vi "AMC Multiple Targets Example 1.vi"() -> ()   [LabVIEW 2013]
uses:
  <vilib>/NI/Tools/Keyed Array/KeyedArray.ctl
  <vilib>/NI/Tools/Keyed Array/Map String.vi
  <vilib>/NI/Tools/String/Get Case Matching.vi
  vi.lib/NI/AMC/AMC.lvlib
  <vilib>/NI/Tools/Keyed Array/Tools_KeyedArray.lvlib
panel:
  out "App Response":string
  in  "request":bool
  in  "App Request":string
  in  "Local UDP Port":u16=8000
  in  "Target UDP Port":u16=9000
  in  "Servers":i32(listbox)
  in  "Get All Queues":bool
  in  "Target IP Address":string="localhost"
  in  "Queue":string
  in  "Verify Queue":bool
  in  "PingAll":bool
  out "Response":string
  in  "Ping":bool
  in  "Remote Exit":bool
  out "Process":bool
  in  "Remote Process":bool
  out "Status":string
  in  "Local Process":bool
  in  "Local Exit":bool
  in  "State Variables":T1
  # "Target 1"
  # "Local Messages >>"
  # "Remote Messages >>"
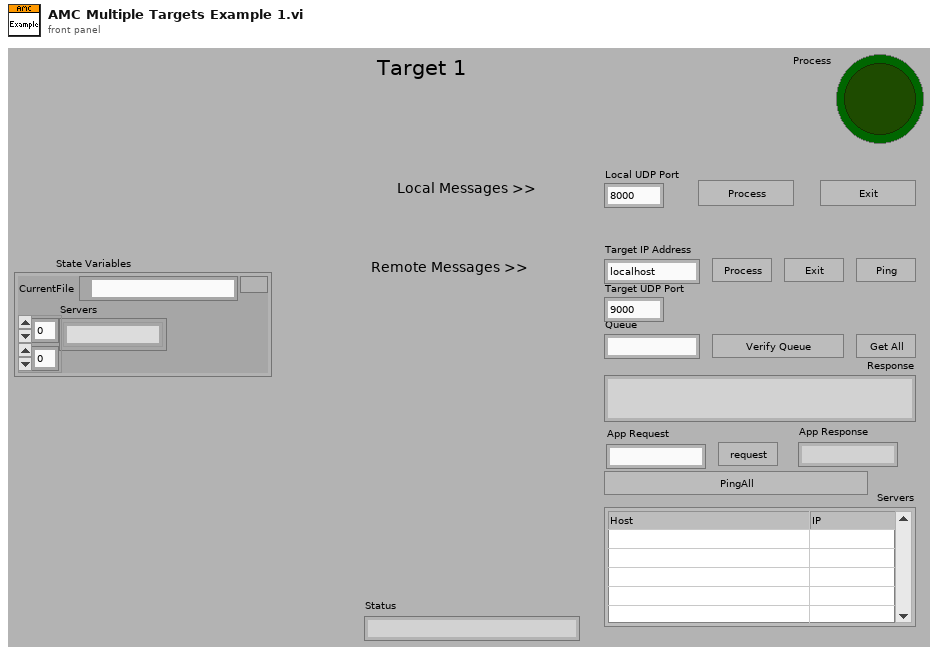
[diagram p1: front panel]
types:
  T1 = cluster{"CurrentFile":path, "Servers":string[][]}
  T2 = typedef "AMC.lvlib/Message Queue.ctl" = refnum<queue>
  T3 = typedef "AMC.lvlib/Message.ctl" = cluster{"name":string, "value":string, "attributes":T4, "receiver host":string, "receiver process":string, "source host":string, "source process":string, "priority message":bool, "acknowledge message":bool}
  T4 = typedef "Tools_KeyedArray.lvlib/KeyedArray.ctl" = cluster{"keys":string[], "values":string[]}
  T5 = typedef "LVPoint32TypeDef.ctl" = cluster{"Horizontal":i32, "Vertical":i32}
  T6 = typedef "LVRowAndColumnTypeDef.ctl" = cluster{"Row":i32, "Column":i32}
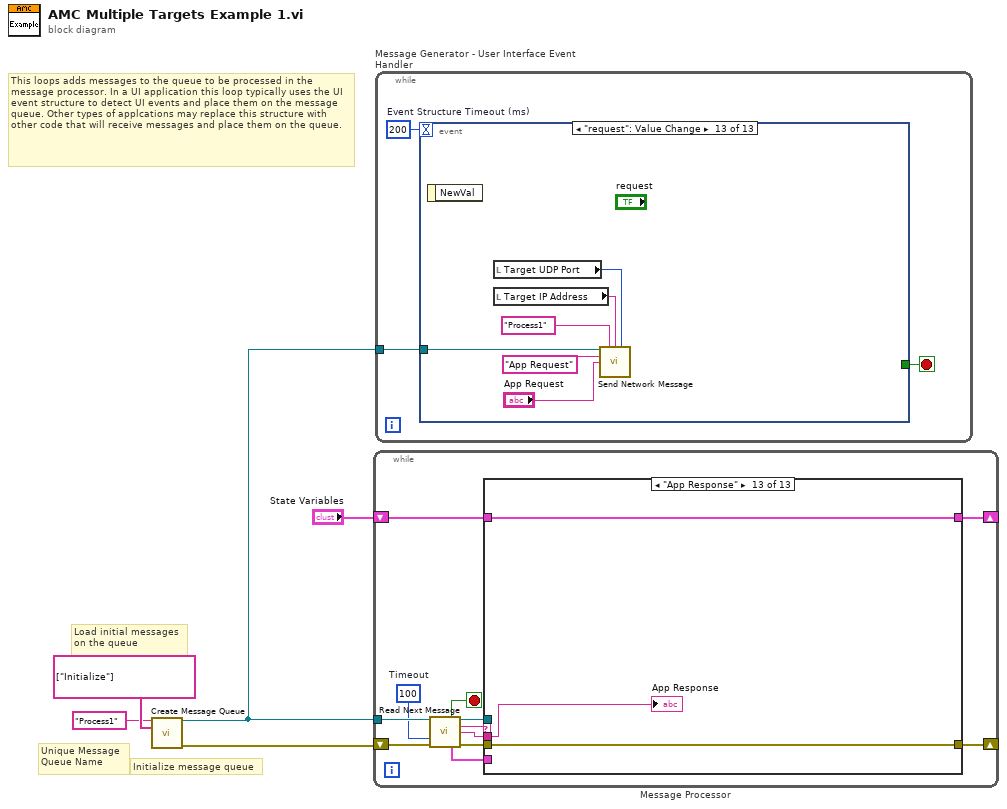
[diagram p0: block diagram]
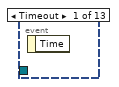
[diagram p2: hidden frame]
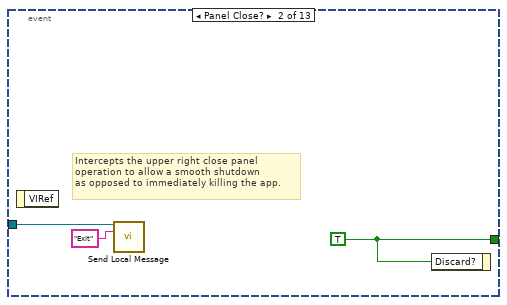
[diagram p3: hidden frame]
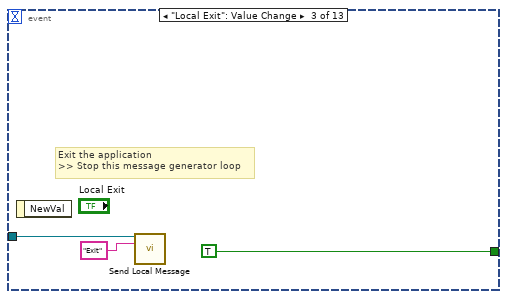
[diagram p4: hidden frame]
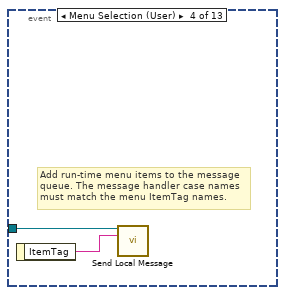
[diagram p5: hidden frame]
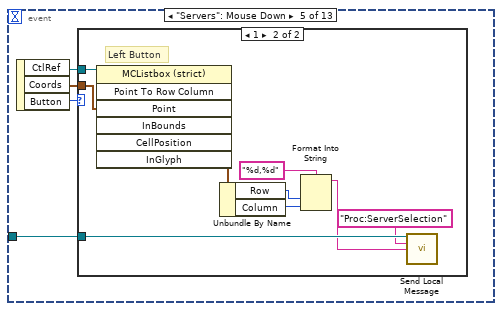
[diagram p6: hidden frame]
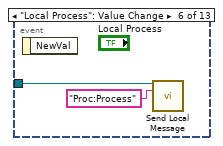
[diagram p8: hidden frame]
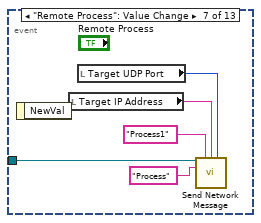
[diagram p9: hidden frame]
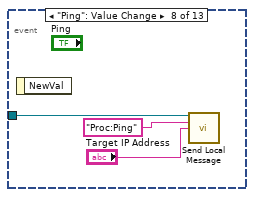
[diagram p10: hidden frame]
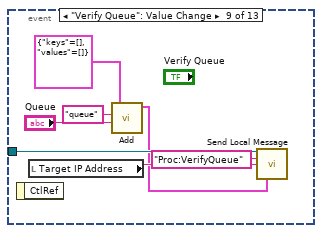
[diagram p11: hidden frame]
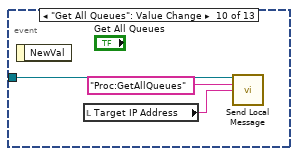
[diagram p12: hidden frame]
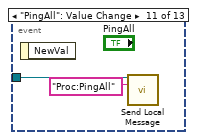
[diagram p13: hidden frame]
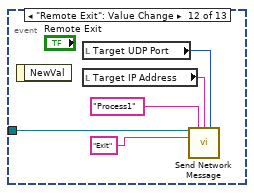
[diagram p14: hidden frame]
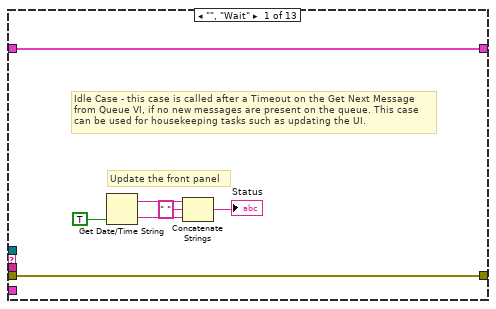
[diagram p15: hidden frame]
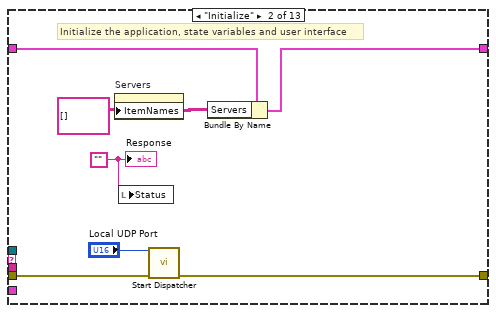
[diagram p16: hidden frame]
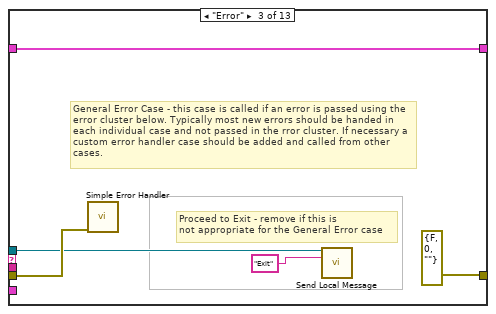
[diagram p17: hidden frame]
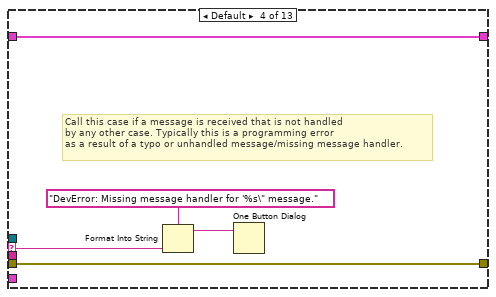
[diagram p18: hidden frame]
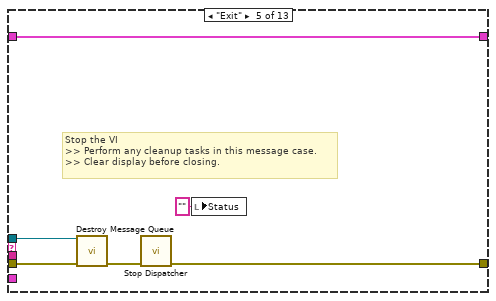
[diagram p19: hidden frame]
diagram:
  # "This loops adds messages to the queue to be processed in the message processor. In a UI application this loop typically uses the UI event structure to detect UI events and place them on the message queue. Other types of applcations may replace this structure with other code that will receive messages and place them on the queue."
  # "Initialize message queue"
  # "Unique Message\nQueue Name"
  # "Load initial messages\non the queue"
  n1 = call "Create Message Queue.vi"("message queue name"="Process1" ("Message queue name (unnamed)"), "initial message names"=string[] ["Initialize"]) -> ("message queue out"=w5:T2, "error out"=w3:errorcluster)  [unwired: 12 in]
  n2 = while "Message Processor" {
    shift-left: w3 -> [w12]
    shift-right: [w13] -> _
    tunnel: w5 -> [w11]
    shift-left: "State Variables" -> [w17]
    shift-right: [w16] -> _
    stop <- w10 stop-if-true
    w6 = 100  # Timeout
    n3 = call "Read Next Message.vi"("message queue in"=w11, "timeout (1 ms)"=w6, "error in"=w12) -> ("exit process?"=w10:bool, "message queue out"=w15:T2, "message name"=w9:string, "message value"=w8:string, "message"=w7:T3, "error out"=w14:errorcluster)  [unwired: 5 in, 2 out]
    n4 = case shown="\"App Response\"" w9 {
      selector: w9 -> [_ _ _ w39 _ _ _ _ _ _ _ _ _]
      tunnel: [w24 w27 w36 w41 w46 w49 w52 w60 w63 w86 w92 w100 w103] -> w16
      tunnel: w17 -> [w24 w28 w36 w41 w46 w49 w52 w60 w64 w86 w92 w100 w103]
      tunnel: w15 -> [_ _ w33 _ w44 _ _ _ _ _ _ _ _]
      tunnel: w14 -> [w23 w30 w34 w40 w47 w48 w53 w59 w69 w80 w89 w99 w101]
      tunnel: [w23 w29 errorcluster {"status"=FALSE, "code"=0, "source"=""} ("error out") w40 w42 w48 w53 w58 w68 w79 w88 w99 w101] -> w13
      tunnel: w7 -> [_ _ _ _ _ _ _ _ _ w85 _ _ _]
      tunnel: w8 -> [_ _ _ _ _ _ _ w56 _ w82 w91 w96 w102]
      frame "", "Wait" {
        # "Update the front panel"
        # "Idle Case - this case is called after a Timeout on the Get Next Message from Queue VI, if no new messages are present on the queue. This case can be used for housekeeping tasks such as updating the UI."
        n5 = Get Date/Time String(want seconds? (F)=TRUE) -> (date string=w22:string, time string=w21:string)  [unwired: 2 out]
        n6 = Concatenate Strings(w22, " " ("string"), w21) -> (→"Status":string)
      }
      frame "Initialize" {
        w26 = string[][] [] ("Item Names")
        w31 = ""
        # "Initialize the application, state variables and user interface"
        n7 = property on="Servers" class="MCListbox (strict)"("ItemNames"=w26) -> ()  [unwired: 2 in, 2 out]
        n8 = local write "Status"(w31) -> ()
        n9 = call "Start Dispatcher.vi"("UDP port (0)"="Local UDP Port", "error in"=w30) -> ("error out"=w29:errorcluster)  [unwired: 11 in, 2 out]
        n10 = Bundle By Name(cluster=w28, "Servers"=w26) -> (w27:T1)
        "Response" <- w31
      }
      frame "Error" {
        # "Proceed to Exit - remove if this is\nnot appropriate for the General Error case"
        # "General Error Case - this case is called if an error is passed using the error cluster below. Typically most new errors should be handed in each individual case and not passed in the rror cluster. If necessary a custom error handler case should be added and called from other cases."
        n11 = call <vilib>:"Simple Error Handler.vi"("error in (no error)"=w34) -> ()  [unwired: 1 in, 8 out]
        n12 = call "Send Local Message.vi"("message queue in"=w33, "message name"="Exit") -> ()  [unwired: 11 in, 3 out]
      }
      frame Default {
        # "Call this case if a message is received that is not handled \nby any other case. Typically this is a programming error\nas a result of a typo or unhandled message/missing message handler."
        n13 = Format Into String(format string="DevError: Missing message handler for '%s\" message." ("message"), w39) -> (resulting string=w37:string)  [unwired: 2 in, 1 out]
        n14 = One Button Dialog(message=w37) -> ()  [unwired: 2 out]
      }
      frame "Exit" {
        # "Stop the VI\n>> Perform any cleanup tasks in this message case.\n>> Clear display before closing."
        n15 = call "Destroy Message Queue.vi"("message queue in"=w44, "error in"=w47) -> ("error out"=w43:errorcluster)  [unwired: 11 in, 2 out]
        n16 = call "Stop Dispatcher.vi"("error in"=w43) -> ("error out"=w42:errorcluster)  [unwired: 14 in]
        n17 = local write "Status"("" ("Status")) -> ()
      }
      frame "**** App Processing Functions ****" {
      }
      frame "Proc:Process" {
        # "Add actions to perform in response to Process button being pressed"
        n18 = feedback #1() -> (w51:bool)  [unwired: 1 out]
        n19 = Not(x=w51) -> (.not. x?=w50:bool)
        "Process" <- w50
        n20 = feedback-in #1(w50) -> ()
      }
      frame "Proc:Ping" {
        n21 = call "Ping Dispatcher.vi"("receiver host (\"\")"=w56, "receiver port (0)"="Target UDP Port", "timeout (100 ms)"=1000 ("Timeout (100 ms)"), "error in"=w59) -> ("string response"=w57:string, "error out"=w58:errorcluster)  [unwired: 9 in, 1 out]
        n22 = local write "Response"(w57) -> ()
      }
      frame "Proc:PingAll" {
        n23 = local read "Target UDP Port"() -> (w61:u16)
        n24 = call "Ping All Dispatchers.vi"("receiver port (0)"=w61, "timeout (1000 ms)"=1000 ("Timeout (1000 ms)"), "error in"=w69) -> ("response messages"=w65:T3[], "response"=w67:string, "error out"=w68:errorcluster)  [unwired: 10 in]
        n25 = for {
          tunnel: w65 -> [w75] mode=indexing
          tunnel: [w70] -> w62 mode=indexing
          n26 = Unbundle By Name(w75) -> ("source host"=w72:string, "attributes"=w74:T4)
          n27 = call <vilib>:"Index.vi"("key"="IP", "array in"=w74) -> ("value"=w71:string)  [unwired: 2 in, 3 out]
          n28 = Build Array(w72, w71) -> (w70:string[])
        }
        n29 = local write "Response"(w67) -> ()
        n30 = property on="Servers" class="MCListbox (strict)"("ItemNames"=w62) -> ()  [unwired: 2 in, 2 out]
        n31 = Bundle By Name(cluster=w64, "Servers"=w62) -> (w63:T1)
      }
      frame "Proc:VerifyQueue" {
        n32 = Unbundle By Name(w85) -> ("attributes"=w84:T4)
        n33 = local read "Target UDP Port"() -> (w76:u16)
        n34 = call <vilib>:"Index.vi"("key"="queue", "array in"=w84) -> ("value"=w77:string)  [unwired: 2 in, 3 out]
        n35 = call "Verify Dispatcher Queue.vi"("receiver host (\"\")"=w82, "receiver port (0)"=w76, "queue name"=w77, "timeout (100 ms)"=1000 ("Timeout (100 ms)"), "error in"=w80) -> ("string response"=w81:string, "error out"=w79:errorcluster)  [unwired: 8 in, 1 out]
        n36 = local write "Response"(w81) -> ()
      }
      frame "Proc:GetAllQueues" {
        n37 = local read "Target UDP Port"() -> (w87:u16)
        n38 = call "Get All Dispatcher Queues.vi"("receiver host (\"\")"=w91, "receiver port (0)"=w87, "error in"=w89) -> ("string response"=w90:string, "error out"=w88:errorcluster)  [unwired: 9 in, 2 out]
        n39 = local write "Response"(w90) -> ()
      }
      frame "Proc:ServerSelection" {
        n40 = Unbundle By Name(w100) -> ("Servers"=w98:string[][])
        n41 = Scan From String(format string="%d,%d", input string=w96) -> (output 1=w94:i32, output 2=w93:i32)  [unwired: 2 in, 5 out]
        n42 = Index Array(array=w98, index (row)=w94, index (col)=w93) -> (element=w97:string)
        n43 = local write "Target IP Address"(w97) -> ()
      }
      frame "App Response" {
        "App Response" <- w102
      }
    }
  }
  n44 = while "Message Generator - User Interface Event Handler" {
    tunnel: w5 -> [w104]
    stop <- w105 stop-if-true
    w106 = 200  # Event Structure Timeout (ms)
    n45 = event shown="[12] \"request\": Value Change" {
      selector: _ -> [_ _ _ _ _ _ _ _ _ _ _ _ _]
      dyn-events: _ -> [_ _ _ _ _ _ _ _ _ _ _ _ _]
      timeout: w106 -> [_ _ _ _ _ _ _ _ _ _ _ _ _]
      tunnel: [_ w109 TRUE ("Discard?") _ _ _ _ _ _ _ _ _ _] -> w105
      tunnel: w104 -> [_ w107 w111 w113 w118 w129 w134 w137 w144 w147 w149 w154 w160]
      event Timeout {
        n46 = event-data() -> ()  [unwired: 2 out]
      }
      event Panel Close? {
        w109 = TRUE ("Discard?")
        # "Intercepts the upper right close panel\noperation to allow a smooth shutdown\nas opposed to immediately killing the app."
        n47 = event-data() -> ()  [unwired: 2 out]
        n48 = call "Send Local Message.vi"("message queue in"=w107, "message name"="Exit") -> ()  [unwired: 11 in, 3 out]
        n49 = event-data("Discard?"=w109) -> ()  [unwired: 1 in, 1 out]
      }
      event "Local Exit": Value Change {
        # "Exit the application\n>> Stop this message generator loop"
        n50 = event-data() -> ()  [unwired: 2 out]
        n51 = call "Send Local Message.vi"("message queue in"=w111, "message name"="Exit") -> ()  [unwired: 11 in, 3 out]
      }
      event Menu Selection (User) {
        # "Add run-time menu items to the message\nqueue. The message handler case names must match the menu ItemTag names."
        n52 = event-data() -> ("ItemTag"=w114:string)  [unwired: 1 out]
        n53 = call "Send Local Message.vi"("message queue in"=w113, "message name"=w114) -> ()  [unwired: 11 in, 3 out]
      }
      event "Servers": Mouse Down {
        n54 = event-data() -> ("CtlRef"=w117:refnum<vi>, "Coords"=w116:T5, "Button"=w115:u16)  [unwired: 1 out]
        n55 = case shown="1" w115 {
          tunnel: w118 -> [_ w127]
          tunnel: w117 -> [_ w125]
          tunnel: w116 -> [_ w124]
          frame Default {
          }
          frame 1 {
            # "Left Button"
            n56 = invoke class="MCListbox (strict)" method="Point To Row Column"(reference=w125, "Point"=w124) -> ("CellPosition"=w123:T6)  [unwired: 5 in, 6 out]
            n57 = Unbundle By Name(w123) -> ("Row"=w122:i32, "Column"=w121:i32)
            n58 = Format Into String(format string="%d,%d", w122, w121) -> (resulting string=w119:string)  [unwired: 2 in, 1 out]
            n59 = call "Send Local Message.vi"("message queue in"=w127, "message name"="Proc:ServerSelection" ("Message Name"), "message value"=w119) -> ()  [unwired: 10 in, 3 out]
          }
        }
      }
      event "Local Process": Value Change {
        n60 = event-data() -> ()  [unwired: 2 out]
        n61 = call "Send Local Message.vi"("message queue in"=w129, "message name"="Proc:Process") -> ()  [unwired: 11 in, 3 out]
      }
      event "Remote Process": Value Change {
        n62 = event-data() -> ()  [unwired: 2 out]
        n63 = local read "Target IP Address"() -> (w131:string)
        n64 = local read "Target UDP Port"() -> (w130:u16)
        n65 = call "Send Network Message.vi"("message queue in"=w134, "receiver process"="Process1" ("process"), "receiver host"=w131, "receiver port (0)"=w130, "message name"="Process") -> ()  [unwired: 8 in, 3 out]
      }
      event "Ping": Value Change {
        n66 = event-data() -> ()  [unwired: 2 out]
        n67 = call "Send Local Message.vi"("message queue in"=w137, "message name"="Proc:Ping" ("Message Name"), "message value"="Target IP Address") -> ()  [unwired: 10 in, 3 out]
      }
      event "Verify Queue": Value Change {
        n68 = event-data() -> ()  [unwired: 2 out]
        n69 = local read "Target IP Address"() -> (w142:string)
        n70 = call <vilib>:"Add.vi"("value"="Queue", "key"="queue", "array in"=T4 {"keys"=[], "values"=[]}) -> ("array out"=w138:T4)  [unwired: 1 in, 3 out]
        n71 = call "Send Local Message.vi"("message queue in"=w144, "message name"="Proc:VerifyQueue" ("Message Name"), "message value"=w142, "message attributes"=w138) -> ()  [unwired: 9 in, 3 out]
      }
      event "Get All Queues": Value Change {
        n72 = event-data() -> ()  [unwired: 2 out]
        n73 = local read "Target IP Address"() -> (w145:string)
        n74 = call "Send Local Message.vi"("message queue in"=w147, "message name"="Proc:GetAllQueues" ("Message Name"), "message value"=w145) -> ()  [unwired: 10 in, 3 out]
      }
      event "PingAll": Value Change {
        n75 = event-data() -> ()  [unwired: 2 out]
        n76 = call "Send Local Message.vi"("message queue in"=w149, "message name"="Proc:PingAll" ("Message Name")) -> ()  [unwired: 11 in, 3 out]
      }
      event "Remote Exit": Value Change {
        n77 = event-data() -> ()  [unwired: 2 out]
        n78 = local read "Target UDP Port"() -> (w150:u16)
        n79 = local read "Target IP Address"() -> (w151:string)
        n80 = call "Send Network Message.vi"("message queue in"=w154, "receiver process"="Process1" ("process"), "receiver host"=w151, "receiver port (0)"=w150, "message name"="Exit") -> ()  [unwired: 8 in, 3 out]
      }
      event "request": Value Change {
        n81 = event-data() -> ()  [unwired: 2 out]
        n82 = local read "Target UDP Port"() -> (w156:u16)
        n83 = local read "Target IP Address"() -> (w157:string)
        n84 = call "Send Network Message.vi"("message queue in"=w160, "receiver process"="Process1" ("process"), "receiver host"=w157, "receiver port (0)"=w156, "message name"="App Request", "message value"="App Request") -> ()  [unwired: 7 in, 3 out]
      }
    }
  }
